vi "PLC_comm.vi"() -> ()   [LabVIEW 2017]
uses:
  <vilib>/addons/database/NI_Database_API.lvlib
  Global/DATA LOG.vi
  Global/Global 1.vi
  <vilib>/DATA AHEAD/SP7/typedefs/PLC Type.ctl
  <vilib>/DATA AHEAD/SP7/SP7.lvlib
  <vilib>/DATA AHEAD/SP7/functions/read/read String.vi
  <vilib>/DATA AHEAD/SP7/functions/write/write Dint array.vi
  <vilib>/DATA AHEAD/SP7/functions/read/read Dint array.vi
  <vilib>/Utility/error.llb/DialogType.ctl
  <vilib>/DATA AHEAD/SP7/functions/read/read real array.vi
  <vilib>/DATA AHEAD/SP7/functions/write/writeString.vi
  <vilib>/addons/database/Connection.llb/DB Tools Open Connec (String).vi
panel:
  out "IP1 7":string
  out "PLC 7":bool
  out "IP1 6":string
  out "PLC 6":bool
  out "IP1 5":string
  out "PLC 5":bool
  out "PLC 4":bool
  out "PLC 3":bool
  out "PLC 2":bool
  out "PLC 1":bool
  out "IP1 4":string
  out "IP1 3":string
  out "IP1 2":string
  out "IP1":string
  in  "stop":bool
  out "error out":errorcluster
  in  "error in (no error)":errorcluster
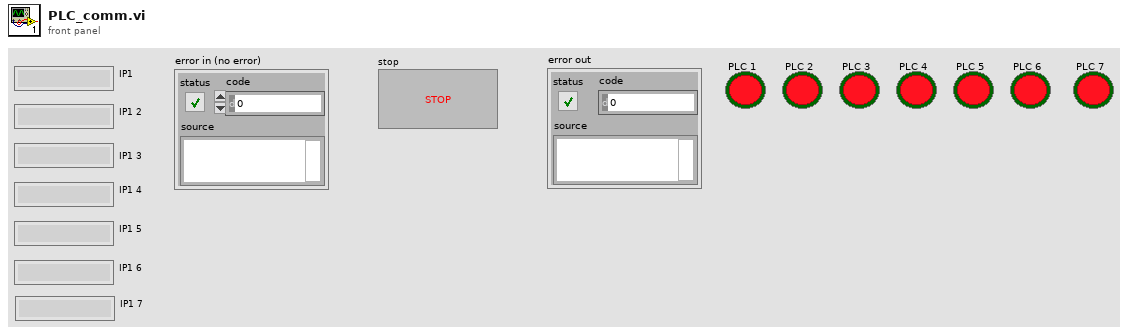
[diagram p1: front panel]
types:
  T1 = typedef "DialogType.ctl" = u16
  T2 = typedef "SP7.lvlib/PLC Type.ctl" = enum16{"S7 200", "S7 300/400", "S7 1200", "S7 1500", "LOGO!8"}
  T3 = typedef "NI_Database_API.lvlib/Conn ObjectReference.ctl" = refnum<k1>
  T4 = typedef "SP7.lvlib/S7 Connection.ctl" = cluster{"TCP Connection Ref":refnum<k5>, "IP address":string, "timeout ms":i32, "Connected?":bool, "PLC Type":T2, "Rack S7 400":u8, "Slot S7 400":u8, "PDU Size":u16, "connection semaphore":T5}
  T5 = typedef "Semaphore RefNum" = refnum<k1>
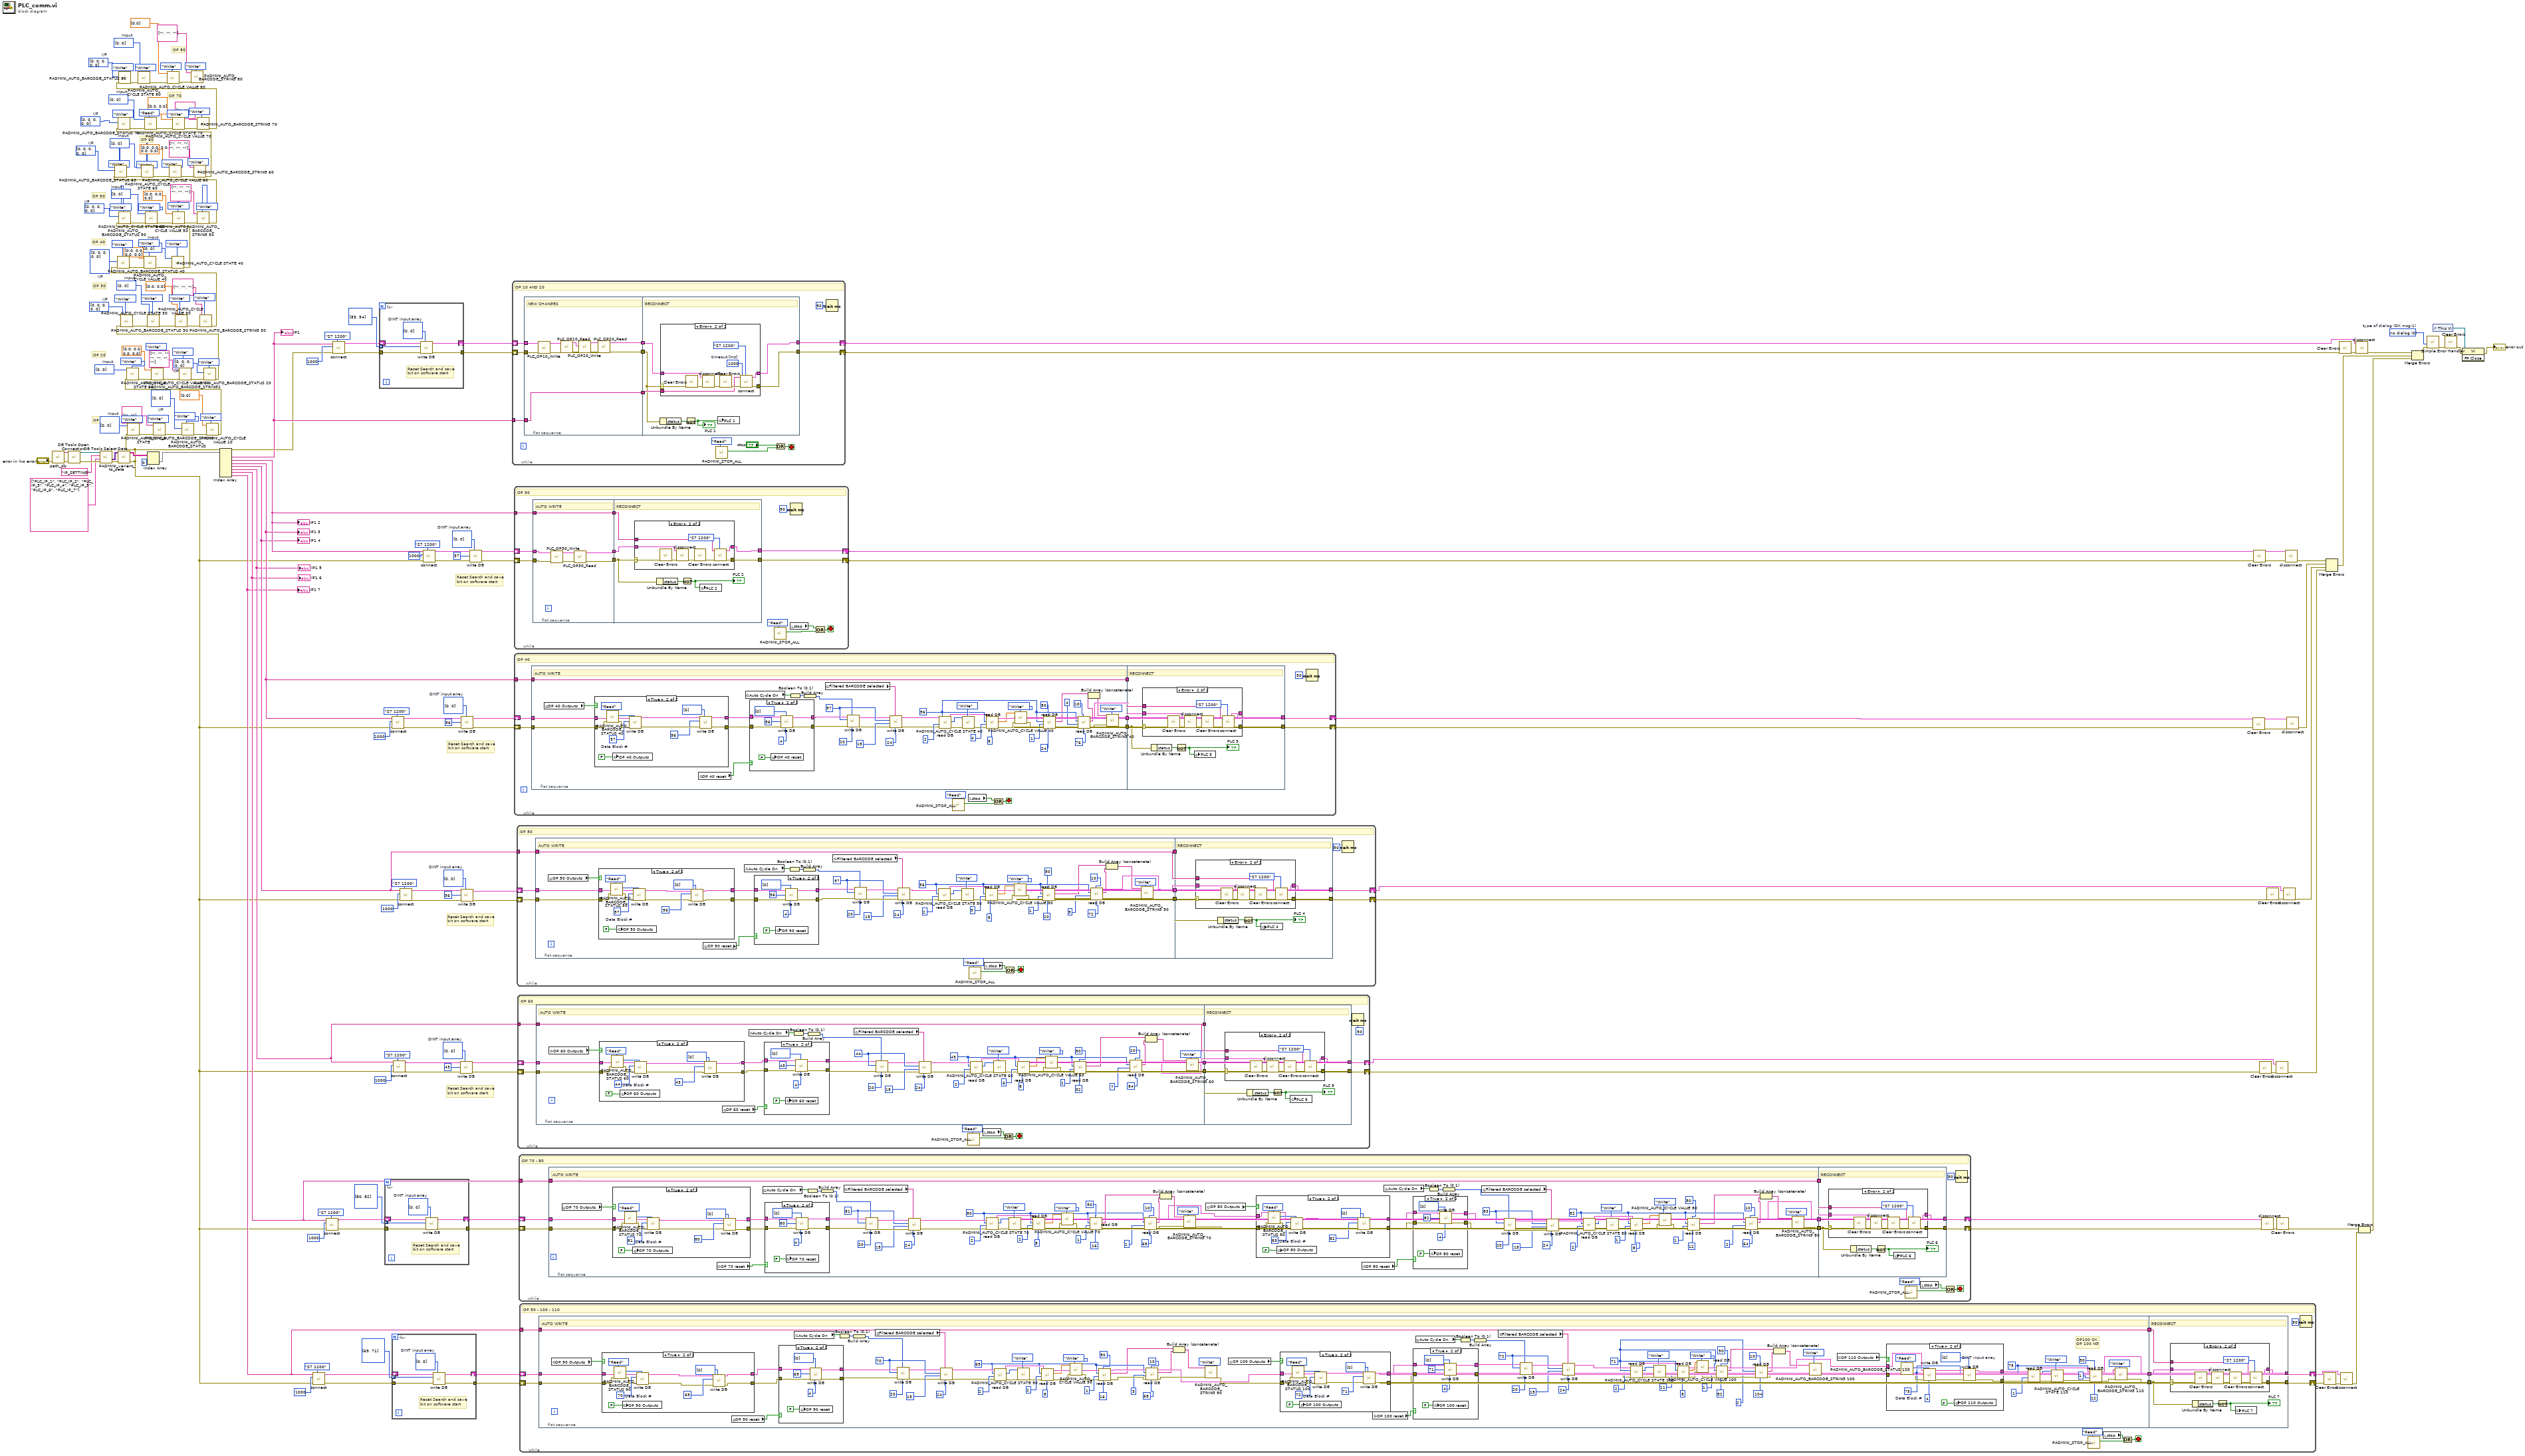
[diagram p0: block diagram]
diagram:
  w15 = i32[] [0, 0]  # DINT input array
  w22 = i32[] [0, 0]  # DINT input array
  w27 = i32[] [0, 0]  # DINT input array
  w39 = i32[] [0, 0]  # DINT input array
  w40 = T1 0 items=["no dialog", "OK message", "continue or stop message", "OK message + warnings", "continue/stop + warnings"]  # type of dialog (OK msg:1)
  w42 = i32[] [0, 0, 0, 0, 0]  # I/P
  w43 = i32[] [0, 0]  # Input
  w45 = i32[] [0, 0]  # Input
  w46 = i32[] [0, 0]  # Input
  w48 = i32[] [0, 0]  # Input
  w44 = i32[] [0, 0, 0, 0, 0]  # I/P
  w47 = i32[] [0, 0, 0, 0, 0]  # I/P
  w49 = i32[] [0, 0, 0, 0, 0]  # I/P
  w50 = i32[] [0, 0, 0, 0, 0]  # I/P
  w51 = i32[] [0, 0]  # Input
  w52 = i32[] [0, 0]  # Input
  w53 = i32[] [0, 0, 0, 0, 0]  # I/P
  w54 = i32[] [0, 0, 0, 0, 0]  # I/P
  w55 = i32[] [0, 0]  # Input
  w56 = i32[] [0, 0]  # I/P
  w57 = i32[] [0, 0]  # Input
  # "Reset Search and save \nbit on software start"
  # "Reset Search and save \nbit on software start"
  # "Reset Search and save \nbit on software start"
  # "Reset Search and save \nbit on software start"
  # "OP 80"
  # "OP 70"
  # "OP 60"
  # "OP 50"
  # "OP 40"
  # "OP 30"
  # "OP 20"
  # "OP 10"
  n1 = call "path_db.vi"("error in"="error in (no error)") -> ("error out"=w196:errorcluster, "resulting string"=w201:string)  [unwired: 9 in]
  n2 = call-poly <vilib>:"DB Tools Open Connection.vi"("error in (no error)"=w196, "connection information"=w201) -> ("error out"=w200:errorcluster, "connection reference"=w199:T3)  [unwired: 6 in]
  n3 = call <vilib>:"DB Tools Select Data.vi"("error in (no error)"=w200, "columns"=string[] ["PLC_IP_1", "PLC_IP_2", "PLC_IP_3", "PLC_IP_4", "PLC_IP_5", "PLC_IP_6", "PLC_IP_7"], "table"="IP_SETTING", "connection reference"=w199) -> ("error out"=w198:errorcluster, "data"=w197:variant[][])  [unwired: 2 in, 1 out]
  n4 = call "PADMINI_varient_to_data.vi"("error in (no error)"=w198, "data"=w197) -> ("error out"=w64:errorcluster, "Array"=w192:string[][])  [unwired: 8 in]
  n5 = call "PADMINI_AUTO_CYCLE STATE.vi"("Enum"=enum16{"Read", "Write"}."Write", "error in (no error)"=w64, "Input"=w57) -> ("error out"=w180:errorcluster)  [unwired: 7 in, 1 out]
  n6 = Index Array(array=w192, index (row)=0) -> (element=w191:string[])  [unwired: 1 in]
  n7 = call "PADMINI_AUTO_BARCODE_STRING.vi"("Enum"=enum16{"Read", "Write"}."Write", "error in (no error)"=w180, "Input"=string[] ["", ""]) -> ("error out"=w177:errorcluster)  [unwired: 7 in, 1 out]
  n8 = call "PADMINI_AUTO_BARCODE_STATUS.vi"("Enum"=enum16{"Read", "Write"}."Write", "error in (no error)"=w177, "I/P"=w56) -> ("error out"=w175:errorcluster)  [unwired: 7 in, 1 out]
  n9 = call "PADMINI_AUTO_CYCLE VALUE 10.vi"("Enum"=enum16{"Read", "Write"}."Write", "error in (no error)"=w175, "Input"=dbl[] [0.0]) -> ("error out"=w169:errorcluster)  [unwired: 7 in, 1 out]
  n10 = call "PADMINI_AUTO_CYCLE STATE 20.vi"("Enum"=enum16{"Read", "Write"}."Write", "error in (no error)"=w169, "Input"=w43) -> ("error out"=w167:errorcluster)  [unwired: 7 in, 1 out]
  n11 = call "PADMINI_AUTO_CYCLE VALUE 20.vi"("Enum"=enum16{"Read", "Write"}."Write", "error in (no error)"=w167, "Input"=dbl[] [0.0, 0.0, 0.0, 0.0]) -> ("error out"=w163:errorcluster)  [unwired: 7 in, 1 out]
  n12 = call "PADMINI_AUTO_BARCODE_STRING2.vi"("Enum"=enum16{"Read", "Write"}."Write", "error in (no error)"=w163, "Input"=string[] ["", "", "", "", "", "", ""]) -> ("error out"=w161:errorcluster)  [unwired: 7 in, 1 out]
  n13 = call "PADMINI_AUTO_BARCODE_STATUS 20.vi"("Enum"=enum16{"Read", "Write"}."Write", "error in (no error)"=w161, "I/P"=w42) -> ("error out"=w157:errorcluster)  [unwired: 7 in, 1 out]
  n14 = call "PADMINI_AUTO_BARCODE_STATUS 30.vi"("Enum"=enum16{"Read", "Write"}."Write", "error in (no error)"=w157, "I/P"=w44) -> ("error out"=w154:errorcluster)  [unwired: 7 in, 1 out]
  n15 = call "PADMINI_AUTO_CYCLE STATE 30.vi"("Enum"=enum16{"Read", "Write"}."Write", "error in (no error)"=w154, "Input"=w45) -> ("error out"=w153:errorcluster)  [unwired: 7 in, 1 out]
  n16 = call "PADMINI_AUTO_CYCLE VALUE 30.vi"("Enum"=enum16{"Read", "Write"}."Write", "error in (no error)"=w153, "Input"=dbl[] [0.0, 0.0]) -> ("error out"=w150:errorcluster)  [unwired: 7 in, 1 out]
  n17 = call "PADMINI_AUTO_BARCODE_STRING 30.vi"("Enum"=enum16{"Read", "Write"}."Write", "error in (no error)"=w150, "Input"=string[] ["", "", ""]) -> ("error out"=w131:errorcluster)  [unwired: 7 in, 1 out]
  n18 = call "PADMINI_AUTO_BARCODE_STATUS 40.vi"("Enum"=enum16{"Read", "Write"}."Write", "error in (no error)"=w131, "I/P"=w47) -> ("error out"=w130:errorcluster)  [unwired: 7 in, 1 out]
  n19 = call "PADMINI_AUTO_CYCLE VALUE 40.vi"("Enum"=enum16{"Read", "Write"}."Write", "error in (no error)"=w130, "Input"=dbl[] [0.0, 0.0, 0.0, 0.0]) -> ("error out"=w129:errorcluster)  [unwired: 7 in, 1 out]
  n20 = call "PADMINI_AUTO_CYCLE STATE 40.vi"("Enum"=enum16{"Read", "Write"}."Write", "error in (no error)"=w129, "Input"=w46) -> ("error out"=w128:errorcluster)  [unwired: 7 in, 1 out]
  n21 = call "PADMINI_AUTO_BARCODE_STATUS 50.vi"("Enum"=enum16{"Read", "Write"}."Write", "error in (no error)"=w128, "I/P"=w49) -> ("error out"=w115:errorcluster)  [unwired: 7 in, 1 out]
  n22 = call "PADMINI_AUTO_CYCLE STATE 50.vi"("Enum"=enum16{"Read", "Write"}."Write", "error in (no error)"=w115, "Input"=w48) -> ("error out"=w119:errorcluster)  [unwired: 7 in, 1 out]
  n23 = call "PADMINI_AUTO_CYCLE VALUE 50.vi"("Enum"=enum16{"Read", "Write"}."Write", "error in (no error)"=w119, "Input"=dbl[] [0.0, 0.0, 0.0]) -> ("error out"=w116:errorcluster)  [unwired: 7 in, 1 out]
  n24 = call "PADMINI_AUTO_BARCODE_STRING 50.vi"("Enum"=enum16{"Read", "Write"}."Write", "error in (no error)"=w116, "Input"=string[] ["", "", "", "", "", ""]) -> ("error out"=w94:errorcluster)  [unwired: 7 in, 1 out]
  n25 = call "PADMINI_AUTO_BARCODE_STATUS 60.vi"("Enum"=enum16{"Read", "Write"}."Write", "error in (no error)"=w94, "I/P"=w50) -> ("error out"=w98:errorcluster)  [unwired: 7 in, 1 out]
  n26 = call "PADMINI_AUTO_CYCLE STATE 60.vi"("Enum"=enum16{"Read", "Write"}."Write", "error in (no error)"=w98, "Input"=w51) -> ("error out"=w100:errorcluster)  [unwired: 7 in, 1 out]
  n27 = call "PADMINI_AUTO_CYCLE VALUE 60.vi"("Enum"=enum16{"Read", "Write"}."Write", "error in (no error)"=w100, "Input"=dbl[] [0.0, 0.0, 0.0, 0.0, 0.0]) -> ("error out"=w103:errorcluster)  [unwired: 7 in, 1 out]
  n28 = call "PADMINI_AUTO_BARCODE_STRING 60.vi"("Enum"=enum16{"Read", "Write"}."Write", "error in (no error)"=w103, "Input"=string[] ["", "", "", "", "", ""]) -> ("error out"=w72:errorcluster)  [unwired: 7 in, 1 out]
  n29 = call "PADMINI_AUTO_BARCODE_STATUS 70.vi"("Enum"=enum16{"Read", "Write"}."Write", "error in (no error)"=w72, "I/P"=w53) -> ("error out"=w75:errorcluster)  [unwired: 7 in, 1 out]
  n30 = call "PADMINI_AUTO_CYCLE STATE 70.vi"("Enum"=enum16{"Read", "Write"}."Read", "error in (no error)"=w75, "Input"=w52) -> ("error out"=w87:errorcluster)  [unwired: 7 in, 1 out]
  n31 = call "PADMINI_AUTO_CYCLE VALUE 70.vi"("Enum"=enum16{"Read", "Write"}."Write", "error in (no error)"=w87, "Input"=dbl[] [0.0, 0.0]) -> ("error out"=w84:errorcluster)  [unwired: 7 in, 1 out]
  n32 = call "PADMINI_AUTO_BARCODE_STRING 70.vi"("Enum"=enum16{"Read", "Write"}."Write", "error in (no error)"=w84, "Input"=string[] ["", ""]) -> ("error out"=w69:errorcluster)  [unwired: 7 in, 1 out]
  n33 = call "PADMINI_AUTO_BARCODE_STATUS 80.vi"("Enum"=enum16{"Read", "Write"}."Write", "error in (no error)"=w69, "I/P"=w54) -> ("error out"=w76:errorcluster)  [unwired: 7 in, 1 out]
  n34 = call "PADMINI_AUTO_CYCLE STATE 80.vi"("Enum"=enum16{"Read", "Write"}."Write", "error in (no error)"=w76, "Input"=w55) -> ("error out"=w80:errorcluster)  [unwired: 7 in, 1 out]
  n35 = call "PADMINI_AUTO_CYCLE VALUE 80.vi"("Enum"=enum16{"Read", "Write"}."Write", "error in (no error)"=w80, "Input"=sgl[] [0.0]) -> ("error out"=w83:errorcluster)  [unwired: 7 in, 1 out]
  n36 = call "PADMINI_AUTO_BARCODE_STRING 80.vi"("Enum"=enum16{"Read", "Write"}."Write", "error in (no error)"=w83, "Input"=string[] ["", "", ""]) -> ()  [unwired: 7 in, 2 out]
  n37 = Index Array(array=w191) -> (element #1=w144:string, element #2=w145:string, element #3=w141:string, element #4=w121:string, element #5=w106:string, element #6=w66:string, element #7=w65:string)  [unwired: 7 in]
  "IP1" <- w144
  "IP1 2" <- w145
  "IP1 3" <- w141
  "IP1 4" <- w121
  "IP1 5" <- w106
  "IP1 6" <- w66
  "IP1 7" <- w65
  n38 = call <vilib>:"connect.vi"("PLC Type"=PLC_Type."S7 1200" ("PLC Type 2"), "error in (no error)"=w64, "timeout [ms]"=1000 ("timeout [ms] 2"), "IP address"=w65) -> ("error out"=w2:errorcluster, "S7 Connection out"=w1:T4)  [unwired: 6 in]
  n39 = call <vilib>:"connect.vi"("PLC Type"=PLC_Type."S7 1200" ("PLC Type 2"), "error in (no error)"=w64, "timeout [ms]"=1000 ("timeout [ms] 2"), "IP address"=w66) -> ("error out"=w6:errorcluster, "S7 Connection out"=w7:T4)  [unwired: 6 in]
  n40 = call <vilib>:"connect.vi"("PLC Type"=PLC_Type."S7 1200" ("PLC Type 2"), "error in (no error)"=w64, "timeout [ms]"=1000, "IP address"=w144) -> ("error out"=w30:errorcluster, "S7 Connection out"=w29:T4)  [unwired: 6 in]
  n41 = for {
    tunnel: u16[] [83, 94] ("Data Block #") -> [w207] mode=indexing
    shift-right: [w205] -> w32
    shift-left: w29 -> [w202]
    tunnel: w30 -> [w203]
    tunnel: [w204] -> w31
    w206 = i32[] [0, 0]  # DINT input array
    # "Reset Search and save \nbit on software start"
    n42 = call-poly <vilib>:"write DB.vi"("DINT input array"=w206, "error in (no error)"=w203, "Data Block #"=w207, "S7 Connection in"=w202) -> ("error out"=w204:errorcluster, "S7 Connection out"=w205:T4)  [unwired: 4 in, 2 out]
  }
  n43 = for {
    tunnel: u16[] [80, 82] ("Data Block #") -> [w213] mode=indexing
    shift-right: [w211] -> w8
    shift-left: w7 -> [w208]
    tunnel: w6 -> [w209]
    tunnel: [w210] -> w9
    w212 = i32[] [0, 0]  # DINT input array
    # "Reset Search and save \nbit on software start"
    n44 = call-poly <vilib>:"write DB.vi"("DINT input array"=w212, "error in (no error)"=w209, "Data Block #"=w213, "S7 Connection in"=w208) -> ("error out"=w210:errorcluster, "S7 Connection out"=w211:T4)  [unwired: 4 in, 2 out]
  }
  n45 = call <vilib>:"connect.vi"("PLC Type"=PLC_Type."S7 1200" ("PLC Type 2"), "error in (no error)"=w64, "timeout [ms]"=1000 ("timeout [ms] 2"), "IP address"=w141) -> ("error out"=w24:errorcluster, "S7 Connection out"=w23:T4)  [unwired: 6 in]
  n46 = for {
    tunnel: u16[] [69, 71] ("Data Block #") -> [w219] mode=indexing
    shift-right: [w217] -> w4
    shift-left: w1 -> [w214]
    tunnel: w2 -> [w215]
    tunnel: [w216] -> w3
    w218 = i32[] [0, 0]  # DINT input array
    # "Reset Search and save \nbit on software start"
    n47 = call-poly <vilib>:"write DB.vi"("DINT input array"=w218, "error in (no error)"=w215, "Data Block #"=w219, "S7 Connection in"=w214) -> ("error out"=w216:errorcluster, "S7 Connection out"=w217:T4)  [unwired: 4 in, 2 out]
  }
  n48 = call <vilib>:"connect.vi"("PLC Type"=PLC_Type."S7 1200" ("PLC Type 2"), "error in (no error)"=w64, "timeout [ms]"=1000 ("timeout [ms] 2"), "IP address"=w106) -> ("error out"=w11:errorcluster, "S7 Connection out"=w12:T4)  [unwired: 6 in]
  n49 = call <vilib>:"connect.vi"("PLC Type"=PLC_Type."S7 1200" ("PLC Type 2"), "error in (no error)"=w64, "timeout [ms]"=1000 ("timeout [ms] 2"), "IP address"=w121) -> ("error out"=w18:errorcluster, "S7 Connection out"=w17:T4)  [unwired: 6 in]
  n50 = call <vilib>:"connect.vi"("PLC Type"=PLC_Type."S7 1200" ("PLC Type 2"), "error in (no error)"=w64, "timeout [ms]"=1000 ("timeout [ms] 2"), "IP address"=w145) -> ("error out"=w36:errorcluster, "S7 Connection out"=w37:T4)  [unwired: 6 in]
  n51 = call-poly <vilib>:"write DB.vi"("DINT input array"=w15, "error in (no error)"=w11, "Data Block #"=u16 43, "S7 Connection in"=w12) -> ("error out"=w14:errorcluster, "S7 Connection out"=w13:T4)  [unwired: 4 in, 2 out]
  n52 = call-poly <vilib>:"write DB.vi"("DINT input array"=w22, "error in (no error)"=w18, "Data Block #"=u16 56, "S7 Connection in"=w17) -> ("error out"=w19:errorcluster, "S7 Connection out"=w20:T4)  [unwired: 4 in, 2 out]
  n53 = call-poly <vilib>:"write DB.vi"("DINT input array"=w27, "error in (no error)"=w24, "Data Block #"=u16 56, "S7 Connection in"=w23) -> ("error out"=w26:errorcluster, "S7 Connection out"=w25:T4)  [unwired: 4 in, 2 out]
  n54 = call-poly <vilib>:"write DB.vi"("DINT input array"=w39, "error in (no error)"=w36, "Data Block #"=u16 37, "S7 Connection in"=w37) -> ("error out"=w35:errorcluster, "S7 Connection out"=w34:T4)  [unwired: 4 in, 2 out]
  n55 = while {
    shift-right: [w222] -> w172
    shift-left: w32 -> [w232]
    shift-right: [w230] -> w185
    shift-left: w31 -> [w231]
    tunnel: w144 -> [w220]
    stop <- w225 stop-if-true
    # "OP 10 AND 20"
    n56 = flat-sequence {
      tunnel: [w235] -> w224
      tunnel: [w241] -> w223
      tunnel: w231 -> [w242]
      tunnel: w232 -> [w243]
      tunnel: [w240] -> w221
      tunnel: w220 -> [w240]
      tunnel: [w247] -> w230
      tunnel: [w246] -> w222
      tunnel: w224 -> [w248]
      tunnel: w223 -> [w244]
      tunnel: w221 -> [w245]
      frame #0 {
        # "NEW CHANGES"
        n57 = call "PLC_OP10_Write.vi"("error in (no error)"=w242, "S7 Connection in"=w243) -> ("error out"=w238:errorcluster, "S7 Connection out"=w239:T4)  [unwired: 8 in]
        n58 = call "PLC_OP10_Read.vi"("error in (no error)"=w238, "S7 Connection in"=w239) -> ("error out"=w237:errorcluster, "S7 Connection out"=w236:T4)  [unwired: 8 in]
        n59 = call "PLC_OP20_Write.vi"("error in (no error)"=w237, "S7 Connection in"=w236) -> ("error out"=w233:errorcluster, "S7 Connection out"=w234:T4)  [unwired: 8 in]
        n60 = call "PLC_OP20_Read.vi"("error in (no error)"=w233, "S7 Connection in"=w234) -> ("error out"=w241:errorcluster, "S7 Connection out 2"=w235:T4)  [unwired: 8 in]
      }
      frame #1 {
        # "RECONNECT"
        n61 = Unbundle By Name(w244) -> ("status"=w250:bool)
        n62 = case shown="Error" w244 {
          selector: w244 -> [w252 w261]
          tunnel: [w251 w258] -> w246
          tunnel: [w252 w259] -> w247
          tunnel: w248 -> [w251 w255]
          tunnel: w245 -> [_ w254]
          frame No Error {
          }
          frame Error {
            w253 = 1000  # timeout [ms]
            n63 = call <vilib>:"Clear Errors.vi"("error in (no error)"=w261) -> ("error out"=w262:errorcluster)  [unwired: 5 in, 1 out]
            n64 = call <vilib>:"disconnect.vi"("error in (no error)"=w262, "S7 Connection in"=w255) -> ("error out"=w260:errorcluster)  [unwired: 8 in, 1 out]
            n65 = call <vilib>:"Clear Errors.vi"("error in (no error)"=w260) -> ("error out"=w257:errorcluster)  [unwired: 5 in, 1 out]
            n66 = call <vilib>:"connect.vi"("PLC Type"=PLC_Type."S7 1200" ("PLC Type 2"), "error in (no error)"=w257, "timeout [ms]"=w253, "IP address"=w254) -> ("error out"=w259:errorcluster, "S7 Connection out"=w258:T4)  [unwired: 6 in]
          }
        }
        n67 = Not(x=w250) -> (.not. x?=w249:bool)
        "PLC 1" <- w249
        n68 = global write "Global 1.vi" "PLC 1"(w249) -> ()
      }
    }
    n69 = call "PADMINI_STOP_ALL.vi"("Enum"=enum16{"Read", "Write"}."Read") -> ("Boolean 2"=w227:bool)  [unwired: 9 in, 1 out]
    n70 = Or(x="stop", y=w227) -> (x .or. y?=w225:bool)
    n71 = Wait (ms)(milliseconds to wait=u32 50) -> ()  [unwired: 1 out]
  }
  n72 = while {
    shift-right: [w265] -> w147
    shift-left: w34 -> [w275]
    shift-right: [w273] -> w146
    shift-left: w35 -> [w274]
    tunnel: w145 -> [w264]
    stop <- w267 stop-if-true
    # "OP 30"
    n73 = flat-sequence {
      tunnel: [w278] -> w271
      tunnel: [w280] -> w266
      tunnel: w274 -> [w282]
      tunnel: w275 -> [w281]
      tunnel: w264 -> [w279]
      tunnel: [w279] -> w263
      tunnel: [w285] -> w273
      tunnel: [w284] -> w265
      tunnel: w271 -> [w287]
      tunnel: w266 -> [w286]
      tunnel: w263 -> [w283]
      frame #0 {
        # "AUTO WRITE"
        n74 = call "PLC_OP30_Write.vi"("error in (no error)"=w282, "S7 Connection in"=w281) -> ("error out"=w276:errorcluster, "S7 Connection out"=w277:T4)  [unwired: 8 in]
        n75 = call "PLC_OP30_Read.vi"("error in (no error)"=w276, "S7 Connection in"=w277) -> ("error out"=w280:errorcluster, "S7 Connection out 2"=w278:T4)  [unwired: 8 in]
      }
      frame #1 {
        # "RECONNECT"
        n76 = case shown="Error" w286 {
          selector: w286 -> [w291 w299]
          tunnel: [w290 w296] -> w284
          tunnel: [w291 w297] -> w285
          tunnel: w287 -> [w290 w293]
          tunnel: w283 -> [_ w292]
          frame No Error {
          }
          frame Error {
            n77 = call <vilib>:"Clear Errors.vi"("error in (no error)"=w299) -> ("error out"=w300:errorcluster)  [unwired: 5 in, 1 out]
            n78 = call <vilib>:"disconnect.vi"("error in (no error)"=w300, "S7 Connection in"=w293) -> ("error out"=w298:errorcluster)  [unwired: 8 in, 1 out]
            n79 = call <vilib>:"Clear Errors.vi"("error in (no error)"=w298) -> ("error out"=w295:errorcluster)  [unwired: 5 in, 1 out]
            n80 = call <vilib>:"connect.vi"("PLC Type"=PLC_Type."S7 1200" ("PLC Type 2"), "error in (no error)"=w295, "IP address"=w292) -> ("error out"=w297:errorcluster, "S7 Connection out"=w296:T4)  [unwired: 7 in]
          }
        }
        n81 = Unbundle By Name(w286) -> ("status"=w289:bool)
        n82 = Not(x=w289) -> (.not. x?=w288:bool)
        "PLC 2" <- w288
        n83 = global write "Global 1.vi" "PLC 2"(w288) -> ()
      }
    }
    n84 = call "PADMINI_STOP_ALL.vi"("Enum"=enum16{"Read", "Write"}."Read") -> ("Boolean 2"=w269:bool)  [unwired: 9 in, 1 out]
    n85 = Wait (ms)(milliseconds to wait=u32 50) -> ()  [unwired: 1 out]
    n86 = local read "stop"() -> (w268:bool)
    n87 = Or(x=w268, y=w269) -> (x .or. y?=w267:bool)
  }
  n88 = while {
    shift-right: [w303] -> w138
    shift-left: w25 -> [w313]
    shift-right: [w311] -> w139
    shift-left: w26 -> [w312]
    tunnel: w141 -> [w302]
    stop <- w305 stop-if-true
    # "OP 40"
    n89 = flat-sequence {
      tunnel: [w325] -> w309
      tunnel: [w344] -> w304
      tunnel: w312 -> [w363]
      tunnel: w313 -> [w362]
      tunnel: w302 -> [w343]
      tunnel: [w343] -> w301
      tunnel: [w391] -> w311
      tunnel: [w390] -> w303
      tunnel: w309 -> [w393]
      tunnel: w304 -> [w392]
      tunnel: w301 -> [w389]
      frame #0 {
        w336 = u16 57 ("Data Block #")
        w324 = u16 56 ("Data Block #")
        # "AUTO WRITE"
        n90 = global read "DATA LOG.vi" "OP 40 Outputs"() -> (w361:bool)
        n91 = case shown="True" w361 {
          tunnel: w362 -> [w374 w387]
          tunnel: [w375 w379] -> w341
          tunnel: [w374 w381] -> w342
          tunnel: w363 -> [w375 w384]
          frame False {
          }
          frame True {
            w388 = u16 57  # Data Block #
            n92 = call "PADMINI_AUTO_BARCODE_STATUS 40.vi"("Enum"=enum16{"Read", "Write"}."Read", "error in (no error)"=w384) -> ("error out"=w383:errorcluster, "O/P"=w385:i32[])  [unwired: 8 in]
            n93 = global write "DATA LOG.vi" "OP 40 Outputs"(FALSE) -> ()
            n94 = call-poly <vilib>:"write DB.vi"("DINT input array"=w385, "error in (no error)"=w383, "Data Block #"=w388, "S7 Connection in"=w387) -> ("error out"=w378:errorcluster, "S7 Connection out"=w380:T4)  [unwired: 4 in, 2 out]
            n95 = call-poly <vilib>:"write DB.vi"("DINT input array"=i32[] [0], "error in (no error)"=w378, "Data Block #"=u16 56, "S7 Connection in"=w380) -> ("error out"=w379:errorcluster, "S7 Connection out"=w381:T4)  [unwired: 4 in, 2 out]
          }
        }
        n96 = global read "DATA LOG.vi" "OP 40 reset"() -> (w340:bool)
        n97 = global read "DATA LOG.vi" "Auto Cycle On"() -> (w316:bool)
        n98 = case shown="True" w340 {
          tunnel: w341 -> [w364 w373]
          tunnel: [w364 w372] -> w329
          tunnel: w342 -> [w365 w371]
          tunnel: [w365 w370] -> w330
          frame False {
          }
          frame True {
            n99 = global write "DATA LOG.vi" "OP 40 reset"(FALSE) -> ()
            n100 = call-poly <vilib>:"write DB.vi"("Item offset [byte]"=u16 4 ("Data Block #"), "DINT input array"=i32[] [0], "error in (no error)"=w373, "Data Block #"=u16 56, "S7 Connection in"=w371) -> ("error out"=w372:errorcluster, "S7 Connection out"=w370:T4)  [unwired: 3 in, 2 out]
          }
        }
        n101 = Boolean To (0,1)(Boolean=w316) -> (0, 1=w315:i16)
        n102 = Build Array(w315) -> (w314:i16[])
        n103 = global read "Global 1.vi" "Filtered BARCODE selected"() -> (w339:string[])
        n104 = call-poly <vilib>:"write DB.vi"("Item offset [byte]"=u32 20, "DINT input array"=w314, "error in (no error)"=w329, "Data Block #"=w336, "S7 Connection in"=w330) -> ("error out"=w334:errorcluster, "S7 Connection out"=w333:T4)  [unwired: 3 in, 2 out]
        n105 = call-poly <vilib>:"write DB.vi"("Item offset [byte]"=u32 24, "Input STRINGS"=w339, "error in (no error)"=w334, "String length reserved in DB (default=254)"=u16 15, "Data Block #"=w336, "S7 Connection in"=w333) -> ("error out"=w331:errorcluster, "S7 Connection out"=w332:T4)  [unwired: 2 in, 2 out]
        n106 = call-poly <vilib>:"read DB.vi"("error in (no error)"=w331, "items #"=u16 2 ("Items # [byte]"), "Data Block #"=w324, "S7 Connection in"=w332) -> ("error out"=w359:errorcluster, "DINT result array"=w357:i32[], "S7 Connection out"=w354:T4)  [unwired: 5 in]
        n107 = call "PADMINI_AUTO_CYCLE STATE 40.vi"("Enum"=enum16{"Read", "Write"}."Write", "error in (no error)"=w359, "Input"=w357) -> ("error out"=w355:errorcluster)  [unwired: 7 in, 1 out]
        n108 = call-poly <vilib>:"read DB.vi"("Item offset [byte]"=u32 8, "error in (no error)"=w355, "items #"=u16 4 ("Items # [byte]"), "Data Block #"=w324, "S7 Connection in"=w354) -> ("error out"=w347:errorcluster, "REAL result array"=w345:sgl[], "S7 Connection out"=w353:T4)  [unwired: 4 in]
        n109 = call "PADMINI_AUTO_CYCLE VALUE 40.vi"("Enum"=enum16{"Read", "Write"}."Write", "error in (no error)"=w347, "Input"=w345) -> ("error out"=w346:errorcluster)  [unwired: 7 in, 1 out]
        n110 = call-poly <vilib>:"read DB.vi"("Item offset [byte]"=u32 24, "String length reserved in DB (default=254)"=u16 50, "error in (no error)"=w346, "items #"=u16 1 ("Items # [byte]"), "Data Block #"=w324, "S7 Connection in"=w353) -> ("error out"=w328:errorcluster, "STRING result Array"=w319:string[], "S7 Connection out"=w326:T4)  [unwired: 2 in, 1 out]
        n111 = call-poly <vilib>:"read DB.vi"("Item offset [byte]"=u32 76, "String length reserved in DB (default=254)"=u16 10, "error in (no error)"=w328, "items #"=u16 4 ("Items # [byte]"), "Data Block #"=w324, "S7 Connection in"=w326) -> ("error out"=w327:errorcluster, "STRING result Array"=w318:string[], "S7 Connection out"=w325:T4)  [unwired: 2 in, 1 out]
        n112 = Build Array (concatenate)(w319, w318) -> (w317:string[])
        n113 = call "PADMINI_AUTO_BARCODE_STRING 40.vi"("Enum"=enum16{"Read", "Write"}."Write", "error in (no error)"=w327, "Input"=w317) -> ("error out"=w344:errorcluster)  [unwired: 7 in, 1 out]
      }
      frame #1 {
        # "RECONNECT"
        n114 = case shown="Error" w392 {
          selector: w392 -> [w397 w405]
          tunnel: [w396 w402] -> w390
          tunnel: [w397 w403] -> w391
          tunnel: w393 -> [w396 w399]
          tunnel: w389 -> [_ w398]
          frame No Error {
          }
          frame Error {
            n115 = call <vilib>:"Clear Errors.vi"("error in (no error)"=w405) -> ("error out"=w406:errorcluster)  [unwired: 5 in, 1 out]
            n116 = call <vilib>:"disconnect.vi"("error in (no error)"=w406, "S7 Connection in"=w399) -> ("error out"=w404:errorcluster)  [unwired: 8 in, 1 out]
            n117 = call <vilib>:"Clear Errors.vi"("error in (no error)"=w404) -> ("error out"=w401:errorcluster)  [unwired: 5 in, 1 out]
            n118 = call <vilib>:"connect.vi"("PLC Type"=PLC_Type."S7 1200" ("PLC Type 2"), "error in (no error)"=w401, "IP address"=w398) -> ("error out"=w403:errorcluster, "S7 Connection out"=w402:T4)  [unwired: 7 in]
          }
        }
        n119 = Unbundle By Name(w392) -> ("status"=w395:bool)
        n120 = Not(x=w395) -> (.not. x?=w394:bool)
        "PLC 3" <- w394
        n121 = global write "Global 1.vi" "PLC 3"(w394) -> ()
      }
    }
    n122 = call "PADMINI_STOP_ALL.vi"("Enum"=enum16{"Read", "Write"}."Read") -> ("Boolean 2"=w307:bool)  [unwired: 9 in, 1 out]
    n123 = local read "stop"() -> (w306:bool)
    n124 = Or(x=w306, y=w307) -> (x .or. y?=w305:bool)
    n125 = Wait (ms)(milliseconds to wait=u32 50) -> ()  [unwired: 1 out]
  }
  n126 = while {
    shift-right: [w409] -> w126
    shift-left: w20 -> [w419]
    shift-right: [w417] -> w125
    shift-left: w19 -> [w418]
    tunnel: w121 -> [w408]
    stop <- w411 stop-if-true
    # "OP 50"
    n127 = flat-sequence {
      tunnel: [w440] -> w415
      tunnel: [w450] -> w410
      tunnel: w418 -> [w469]
      tunnel: w419 -> [w468]
      tunnel: w408 -> [w449]
      tunnel: [w449] -> w407
      tunnel: [w497] -> w417
      tunnel: [w496] -> w409
      tunnel: w415 -> [w499]
      tunnel: w410 -> [w498]
      tunnel: w407 -> [w495]
      frame #0 {
        w431 = u16 57 ("Data Block #")
        w439 = u16 56 ("Data Block #")
        # "AUTO WRITE"
        n128 = global read "DATA LOG.vi" "OP 50 Outputs"() -> (w467:bool)
        n129 = case shown="True" w467 {
          tunnel: w468 -> [w480 w493]
          tunnel: [w481 w482] -> w448
          tunnel: [w480 w485] -> w447
          tunnel: w469 -> [w481 w490]
          frame False {
          }
          frame True {
            w494 = u16 57  # Data Block #
            n130 = call "PADMINI_AUTO_BARCODE_STATUS 50.vi"("Enum"=enum16{"Read", "Write"}."Read", "error in (no error)"=w490) -> ("error out"=w489:errorcluster, "O/P"=w491:i32[])  [unwired: 8 in]
            n131 = global write "DATA LOG.vi" "OP 50 Outputs"(FALSE) -> ()
            n132 = call-poly <vilib>:"write DB.vi"("DINT input array"=w491, "error in (no error)"=w489, "Data Block #"=w494, "S7 Connection in"=w493) -> ("error out"=w483:errorcluster, "S7 Connection out"=w484:T4)  [unwired: 4 in, 2 out]
            n133 = call-poly <vilib>:"write DB.vi"("DINT input array"=i32[] [0] ("Data Byte"), "error in (no error)"=w483, "Data Block #"=u16 56, "S7 Connection in"=w484) -> ("error out"=w482:errorcluster, "S7 Connection out"=w485:T4)  [unwired: 4 in, 2 out]
          }
        }
        n134 = global read "DATA LOG.vi" "OP 50 reset"() -> (w446:bool)
        n135 = global read "DATA LOG.vi" "Auto Cycle On"() -> (w422:bool)
        n136 = case shown="True" w446 {
          tunnel: w448 -> [w470 w479]
          tunnel: [w470 w478] -> w424
          tunnel: w447 -> [w471 w477]
          tunnel: [w471 w476] -> w427
          frame False {
          }
          frame True {
            n137 = global write "DATA LOG.vi" "OP 50 reset"(FALSE) -> ()
            n138 = call-poly <vilib>:"write DB.vi"("Item offset [byte]"=u16 4 ("Data Block #"), "DINT input array"=i32[] [0], "error in (no error)"=w479, "Data Block #"=u16 56, "S7 Connection in"=w477) -> ("error out"=w478:errorcluster, "S7 Connection out"=w476:T4)  [unwired: 3 in, 2 out]
          }
        }
        n139 = Boolean To (0,1)(Boolean=w422) -> (0, 1=w421:i16)
        n140 = Build Array(w421) -> (w420:i16[])
        n141 = global read "Global 1.vi" "Filtered BARCODE selected"() -> (w428:string[])
        n142 = call-poly <vilib>:"write DB.vi"("Item offset [byte]"=u32 20, "DINT input array"=w420, "error in (no error)"=w424, "Data Block #"=w431, "S7 Connection in"=w427) -> ("error out"=w433:errorcluster, "S7 Connection out"=w434:T4)  [unwired: 3 in, 2 out]
        n143 = call-poly <vilib>:"write DB.vi"("Item offset [byte]"=u32 24, "Input STRINGS"=w428, "error in (no error)"=w433, "String length reserved in DB (default=254)"=u16 15, "Data Block #"=w431, "S7 Connection in"=w434) -> ("error out"=w425:errorcluster, "S7 Connection out"=w426:T4)  [unwired: 2 in, 2 out]
        n144 = call-poly <vilib>:"read DB.vi"("error in (no error)"=w425, "items #"=u16 2 ("Items # [byte]"), "Data Block #"=w439, "S7 Connection in"=w426) -> ("error out"=w465:errorcluster, "DINT result array"=w463:i32[], "S7 Connection out"=w460:T4)  [unwired: 5 in]
        n145 = call "PADMINI_AUTO_CYCLE STATE 50.vi"("Enum"=enum16{"Read", "Write"}."Write", "error in (no error)"=w465, "Input"=w463) -> ("error out"=w461:errorcluster)  [unwired: 7 in, 1 out]
        n146 = call-poly <vilib>:"read DB.vi"("Item offset [byte]"=u32 8, "error in (no error)"=w461, "items #"=u16 3 ("Items # [byte]"), "Data Block #"=w439, "S7 Connection in"=w460) -> ("error out"=w453:errorcluster, "REAL result array"=w451:sgl[], "S7 Connection out"=w459:T4)  [unwired: 4 in]
        n147 = call "PADMINI_AUTO_CYCLE VALUE 50.vi"("Enum"=enum16{"Read", "Write"}."Write", "error in (no error)"=w453, "Input"=w451) -> ("error out"=w452:errorcluster)  [unwired: 7 in, 1 out]
        n148 = call-poly <vilib>:"read DB.vi"("Item offset [byte]"=u32 20, "String length reserved in DB (default=254)"=u16 50, "error in (no error)"=w452, "items #"=u16 1 ("Items # [byte]"), "Data Block #"=w439, "S7 Connection in"=w459) -> ("error out"=w442:errorcluster, "STRING result Array"=w438:string[], "S7 Connection out"=w441:T4)  [unwired: 2 in, 1 out]
        n149 = call-poly <vilib>:"read DB.vi"("Item offset [byte]"=u32 72, "String length reserved in DB (default=254)"=u16 10, "error in (no error)"=w442, "items #"=u16 5 ("Items # [byte]"), "Data Block #"=w439, "S7 Connection in"=w441) -> ("error out"=w443:errorcluster, "STRING result Array"=w437:string[], "S7 Connection out"=w440:T4)  [unwired: 2 in, 1 out]
        n150 = Build Array (concatenate)(w438, w437) -> (w436:string[])
        n151 = call "PADMINI_AUTO_BARCODE_STRING 50.vi"("Enum"=enum16{"Read", "Write"}."Write", "error in (no error)"=w443, "Input"=w436) -> ("error out"=w450:errorcluster)  [unwired: 7 in, 1 out]
      }
      frame #1 {
        # "RECONNECT"
        n152 = case shown="Error" w498 {
          selector: w498 -> [w503 w511]
          tunnel: [w502 w508] -> w496
          tunnel: [w503 w509] -> w497
          tunnel: w499 -> [w502 w505]
          tunnel: w495 -> [_ w504]
          frame No Error {
          }
          frame Error {
            n153 = call <vilib>:"Clear Errors.vi"("error in (no error)"=w511) -> ("error out"=w512:errorcluster)  [unwired: 5 in, 1 out]
            n154 = call <vilib>:"disconnect.vi"("error in (no error)"=w512, "S7 Connection in"=w505) -> ("error out"=w510:errorcluster)  [unwired: 8 in, 1 out]
            n155 = call <vilib>:"Clear Errors.vi"("error in (no error)"=w510) -> ("error out"=w507:errorcluster)  [unwired: 5 in, 1 out]
            n156 = call <vilib>:"connect.vi"("PLC Type"=PLC_Type."S7 1200" ("PLC Type 2"), "error in (no error)"=w507, "IP address"=w504) -> ("error out"=w509:errorcluster, "S7 Connection out"=w508:T4)  [unwired: 7 in]
          }
        }
        n157 = Unbundle By Name(w498) -> ("status"=w501:bool)
        n158 = Not(x=w501) -> (.not. x?=w500:bool)
        "PLC 4" <- w500
        n159 = global write "Global 1.vi" "PLC 4"(w500) -> ()
      }
    }
    n160 = call "PADMINI_STOP_ALL.vi"("Enum"=enum16{"Read", "Write"}."Read") -> ("Boolean 2"=w413:bool)  [unwired: 9 in, 1 out]
    n161 = local read "stop"() -> (w412:bool)
    n162 = Or(x=w412, y=w413) -> (x .or. y?=w411:bool)
    n163 = Wait (ms)(milliseconds to wait=u32 50) -> ()  [unwired: 1 out]
  }
  n164 = while {
    shift-right: [w515] -> w107
    shift-left: w13 -> [w525]
    shift-right: [w523] -> w108
    shift-left: w14 -> [w524]
    tunnel: w106 -> [w514]
    stop <- w517 stop-if-true
    # "OP 60"
    n165 = flat-sequence {
      tunnel: [w534] -> w521
      tunnel: [w556] -> w516
      tunnel: w524 -> [w575]
      tunnel: w525 -> [w574]
      tunnel: w514 -> [w555]
      tunnel: [w555] -> w513
      tunnel: [w603] -> w523
      tunnel: [w602] -> w515
      tunnel: w521 -> [w605]
      tunnel: w516 -> [w604]
      tunnel: w513 -> [w601]
      frame #0 {
        w551 = u16 44 ("Data Block #")
        w531 = u16 43 ("Data Block #")
        # "AUTO WRITE"
        n166 = global read "DATA LOG.vi" "OP 60 Outputs"() -> (w573:bool)
        n167 = case shown="True" w573 {
          tunnel: w574 -> [w586 w599]
          tunnel: [w587 w588] -> w543
          tunnel: [w586 w591] -> w542
          tunnel: w575 -> [w587 w596]
          frame False {
          }
          frame True {
            w600 = u16 44  # Data Block #
            n168 = call "PADMINI_AUTO_BARCODE_STATUS 60.vi"("Enum"=enum16{"Read", "Write"}."Read", "error in (no error)"=w596) -> ("error out"=w595:errorcluster, "O/P"=w597:i32[])  [unwired: 8 in]
            n169 = global write "DATA LOG.vi" "OP 60 Outputs"(FALSE) -> ()
            n170 = call-poly <vilib>:"write DB.vi"("DINT input array"=w597, "error in (no error)"=w595, "Data Block #"=w600, "S7 Connection in"=w599) -> ("error out"=w589:errorcluster, "S7 Connection out"=w590:T4)  [unwired: 4 in, 2 out]
            n171 = call-poly <vilib>:"write DB.vi"("DINT input array"=i32[] [0] ("Data Byte"), "error in (no error)"=w589, "Data Block #"=u16 43, "S7 Connection in"=w590) -> ("error out"=w588:errorcluster, "S7 Connection out"=w591:T4)  [unwired: 4 in, 2 out]
          }
        }
        n172 = global read "DATA LOG.vi" "OP 60 reset"() -> (w541:bool)
        n173 = global read "DATA LOG.vi" "Auto Cycle On"() -> (w528:bool)
        n174 = case shown="True" w541 {
          tunnel: w543 -> [w576 w585]
          tunnel: [w576 w584] -> w544
          tunnel: w542 -> [w577 w583]
          tunnel: [w577 w582] -> w545
          frame False {
          }
          frame True {
            n175 = global write "DATA LOG.vi" "OP 60 reset"(FALSE) -> ()
            n176 = call-poly <vilib>:"write DB.vi"("Item offset [byte]"=u16 4 ("Data Block #"), "DINT input array"=i32[] [0], "error in (no error)"=w585, "Data Block #"=u16 43, "S7 Connection in"=w583) -> ("error out"=w584:errorcluster, "S7 Connection out"=w582:T4)  [unwired: 3 in, 2 out]
          }
        }
        n177 = Boolean To (0,1)(Boolean=w528) -> (0, 1=w527:i16)
        n178 = Build Array(w527) -> (w526:i16[])
        n179 = global read "Global 1.vi" "Filtered BARCODE selected"() -> (w554:string[])
        n180 = call-poly <vilib>:"write DB.vi"("Item offset [byte]"=u32 20, "DINT input array"=w526, "error in (no error)"=w544, "Data Block #"=w551, "S7 Connection in"=w545) -> ("error out"=w549:errorcluster, "S7 Connection out"=w548:T4)  [unwired: 3 in, 2 out]
        n181 = call-poly <vilib>:"write DB.vi"("Item offset [byte]"=u32 24, "Input STRINGS"=w554, "error in (no error)"=w549, "String length reserved in DB (default=254)"=u16 15, "Data Block #"=w551, "S7 Connection in"=w548) -> ("error out"=w546:errorcluster, "S7 Connection out"=w547:T4)  [unwired: 2 in, 2 out]
        n182 = call-poly <vilib>:"read DB.vi"("error in (no error)"=w546, "items #"=u16 2 ("Items # [byte]"), "Data Block #"=w531, "S7 Connection in"=w547) -> ("error out"=w571:errorcluster, "DINT result array"=w569:i32[], "S7 Connection out"=w566:T4)  [unwired: 5 in]
        n183 = call "PADMINI_AUTO_CYCLE STATE 60.vi"("Enum"=enum16{"Read", "Write"}."Write", "error in (no error)"=w571, "Input"=w569) -> ("error out"=w567:errorcluster)  [unwired: 7 in, 1 out]
        n184 = call-poly <vilib>:"read DB.vi"("Item offset [byte]"=u32 8, "error in (no error)"=w567, "items #"=u16 6 ("Items # [byte]"), "Data Block #"=w531, "S7 Connection in"=w566) -> ("error out"=w559:errorcluster, "REAL result array"=w557:sgl[], "S7 Connection out"=w565:T4)  [unwired: 4 in]
        n185 = call "PADMINI_AUTO_CYCLE VALUE 60.vi"("Enum"=enum16{"Read", "Write"}."Write", "error in (no error)"=w559, "Input"=w557) -> ("error out"=w558:errorcluster)  [unwired: 7 in, 1 out]
        n186 = call-poly <vilib>:"read DB.vi"("Item offset [byte]"=u32 32, "String length reserved in DB (default=254)"=u16 50, "error in (no error)"=w558, "items #"=u16 1 ("Items # [byte]"), "Data Block #"=w531, "S7 Connection in"=w565) -> ("error out"=w536:errorcluster, "STRING result Array"=w533:string[], "S7 Connection out"=w535:T4)  [unwired: 2 in, 1 out]
        n187 = call-poly <vilib>:"read DB.vi"("Item offset [byte]"=u32 84, "String length reserved in DB (default=254)"=u16 10, "error in (no error)"=w536, "items #"=u16 7 ("Items # [byte]"), "Data Block #"=w531, "S7 Connection in"=w535) -> ("error out"=w537:errorcluster, "STRING result Array"=w540:string[], "S7 Connection out"=w534:T4)  [unwired: 2 in, 1 out]
        n188 = Build Array (concatenate)(w533, w540) -> (w532:string[])
        n189 = call "PADMINI_AUTO_BARCODE_STRING 60.vi"("Enum"=enum16{"Read", "Write"}."Write", "error in (no error)"=w537, "Input"=w532) -> ("error out"=w556:errorcluster)  [unwired: 7 in, 1 out]
      }
      frame #1 {
        # "RECONNECT"
        n190 = case shown="Error" w604 {
          selector: w604 -> [w609 w617]
          tunnel: [w608 w614] -> w602
          tunnel: [w609 w615] -> w603
          tunnel: w605 -> [w608 w611]
          tunnel: w601 -> [_ w610]
          frame No Error {
          }
          frame Error {
            n191 = call <vilib>:"Clear Errors.vi"("error in (no error)"=w617) -> ("error out"=w618:errorcluster)  [unwired: 5 in, 1 out]
            n192 = call <vilib>:"disconnect.vi"("error in (no error)"=w618, "S7 Connection in"=w611) -> ("error out"=w616:errorcluster)  [unwired: 8 in, 1 out]
            n193 = call <vilib>:"Clear Errors.vi"("error in (no error)"=w616) -> ("error out"=w613:errorcluster)  [unwired: 5 in, 1 out]
            n194 = call <vilib>:"connect.vi"("PLC Type"=PLC_Type."S7 1200" ("PLC Type 2"), "error in (no error)"=w613, "IP address"=w610) -> ("error out"=w615:errorcluster, "S7 Connection out"=w614:T4)  [unwired: 7 in]
          }
        }
        n195 = Unbundle By Name(w604) -> ("status"=w607:bool)
        n196 = Not(x=w607) -> (.not. x?=w606:bool)
        "PLC 5" <- w606
        n197 = global write "Global 1.vi" "PLC 5"(w606) -> ()
      }
    }
    n198 = call "PADMINI_STOP_ALL.vi"("Enum"=enum16{"Read", "Write"}."Read") -> ("Boolean 2"=w519:bool)  [unwired: 9 in, 1 out]
    n199 = local read "stop"() -> (w518:bool)
    n200 = Or(x=w518, y=w519) -> (x .or. y?=w517:bool)
    n201 = Wait (ms)(milliseconds to wait=u32 50) -> ()  [unwired: 1 out]
  }
  n202 = while {
    shift-right: [w621] -> w89
    shift-left: w8 -> [w631]
    shift-right: [w629] -> w90
    shift-left: w9 -> [w630]
    tunnel: w66 -> [w620]
    stop <- w623 stop-if-true
    # "OP 70 - 80"
    n203 = flat-sequence {
      tunnel: [w642] -> w627
      tunnel: [w690] -> w622
      tunnel: w630 -> [w728]
      tunnel: w631 -> [w727]
      tunnel: w620 -> [w709]
      tunnel: [w709] -> w619
      tunnel: [w781] -> w629
      tunnel: [w780] -> w621
      tunnel: w627 -> [w783]
      tunnel: w622 -> [w782]
      tunnel: w619 -> [w779]
      frame #0 {
        w658 = u16 83 ("Data Block #")
        w683 = u16 81 ("Data Block #")
        w641 = u16 82 ("Data Block #")
        w664 = u16 80 ("Data Block #")
        # "AUTO WRITE"
        n204 = global read "DATA LOG.vi" "OP 70 Outputs"() -> (w726:bool)
        n205 = case shown="True" w726 {
          tunnel: w727 -> [w764 w777]
          tunnel: [w765 w768] -> w688
          tunnel: [w764 w769] -> w687
          tunnel: w728 -> [w765 w774]
          frame False {
          }
          frame True {
            w778 = u16 81  # Data Block #
            n206 = call "PADMINI_AUTO_BARCODE_STATUS 70.vi"("Enum"=enum16{"Read", "Write"}."Read", "error in (no error)"=w774) -> ("error out"=w773:errorcluster, "O/P"=w775:i32[])  [unwired: 8 in]
            n207 = global write "DATA LOG.vi" "OP 70 Outputs"(FALSE) -> ()
            n208 = call-poly <vilib>:"write DB.vi"("DINT input array"=w775, "error in (no error)"=w773, "Data Block #"=w778, "S7 Connection in"=w777) -> ("error out"=w766:errorcluster, "S7 Connection out"=w767:T4)  [unwired: 4 in, 2 out]
            n209 = call-poly <vilib>:"write DB.vi"("DINT input array"=i32[] [0] ("Data Byte"), "error in (no error)"=w766, "Data Block #"=u16 80, "S7 Connection in"=w767) -> ("error out"=w768:errorcluster, "S7 Connection out"=w769:T4)  [unwired: 4 in, 2 out]
          }
        }
        n210 = global read "DATA LOG.vi" "OP 70 reset"() -> (w689:bool)
        n211 = global read "DATA LOG.vi" "Auto Cycle On"() -> (w634:bool)
        n212 = case shown="True" w689 {
          tunnel: w688 -> [w739 w748]
          tunnel: [w739 w747] -> w678
          tunnel: w687 -> [w740 w746]
          tunnel: [w740 w745] -> w679
          frame False {
          }
          frame True {
            n213 = global write "DATA LOG.vi" "OP 70 reset"(FALSE) -> ()
            n214 = call-poly <vilib>:"write DB.vi"("Item offset [byte]"=u16 4 ("Data Block #"), "DINT input array"=i32[] [0], "error in (no error)"=w748, "Data Block #"=u16 80, "S7 Connection in"=w746) -> ("error out"=w747:errorcluster, "S7 Connection out"=w745:T4)  [unwired: 3 in, 2 out]
          }
        }
        n215 = Boolean To (0,1)(Boolean=w634) -> (0, 1=w633:i16)
        n216 = Build Array(w633) -> (w632:i16[])
        n217 = global read "Global 1.vi" "Filtered BARCODE selected"() -> (w680:string[])
        n218 = call-poly <vilib>:"write DB.vi"("Item offset [byte]"=u32 20, "DINT input array"=w632, "error in (no error)"=w678, "Data Block #"=w683, "S7 Connection in"=w679) -> ("error out"=w685:errorcluster, "S7 Connection out"=w686:T4)  [unwired: 3 in, 2 out]
        n219 = call-poly <vilib>:"write DB.vi"("Item offset [byte]"=u32 24, "Input STRINGS"=w680, "error in (no error)"=w685, "String length reserved in DB (default=254)"=u16 15, "Data Block #"=w683, "S7 Connection in"=w686) -> ("error out"=w676:errorcluster, "S7 Connection out"=w677:T4)  [unwired: 2 in, 2 out]
        n220 = call-poly <vilib>:"read DB.vi"("error in (no error)"=w676, "items #"=u16 2 ("Items # [byte]"), "Data Block #"=w664, "S7 Connection in"=w677) -> ("error out"=w724:errorcluster, "DINT result array"=w722:i32[], "S7 Connection out"=w719:T4)  [unwired: 5 in]
        n221 = call "PADMINI_AUTO_CYCLE STATE 70.vi"("Enum"=enum16{"Read", "Write"}."Write", "error in (no error)"=w724, "Input"=w722) -> ("error out"=w720:errorcluster)  [unwired: 7 in, 1 out]
        n222 = call-poly <vilib>:"read DB.vi"("Item offset [byte]"=u32 8, "error in (no error)"=w720, "items #"=u16 2 ("Items # [byte]"), "Data Block #"=w664, "S7 Connection in"=w719) -> ("error out"=w712:errorcluster, "REAL result array"=w710:sgl[], "S7 Connection out"=w718:T4)  [unwired: 4 in]
        n223 = call "PADMINI_AUTO_CYCLE VALUE 70.vi"("Enum"=enum16{"Read", "Write"}."Write", "error in (no error)"=w712, "Input"=w710) -> ("error out"=w711:errorcluster)  [unwired: 7 in, 1 out]
        n224 = call-poly <vilib>:"read DB.vi"("Item offset [byte]"=u32 16, "String length reserved in DB (default=254)"=u16 50, "error in (no error)"=w711, "items #"=u16 1 ("Items # [byte]"), "Data Block #"=w664, "S7 Connection in"=w718) -> ("error out"=w669:errorcluster, "STRING result Array"=w668:string[], "S7 Connection out"=w670:T4)  [unwired: 2 in, 1 out]
        n225 = call-poly <vilib>:"read DB.vi"("Item offset [byte]"=u32 68, "String length reserved in DB (default=254)"=u16 10, "error in (no error)"=w669, "items #"=u16 1 ("Items # [byte]"), "Data Block #"=w664, "S7 Connection in"=w670) -> ("error out"=w671:errorcluster, "STRING result Array"=w672:string[], "S7 Connection out"=w665:T4)  [unwired: 2 in, 1 out]
        n226 = Build Array (concatenate)(w668, w672) -> (w666:string[])
        n227 = call "PADMINI_AUTO_BARCODE_STRING 70.vi"("Enum"=enum16{"Read", "Write"}."Write", "error in (no error)"=w671, "Input"=w666) -> ("error out"=w691:errorcluster)  [unwired: 7 in, 1 out]
        n228 = global read "DATA LOG.vi" "OP 80 Outputs"() -> (w692:bool)
        n229 = case shown="True" w692 {
          tunnel: [w750 w753] -> w663
          tunnel: [w749 w754] -> w639
          tunnel: w691 -> [w750 w760]
          tunnel: w665 -> [w749 w757]
          frame False {
          }
          frame True {
            w763 = u16 83  # Data Block #
            n230 = call "PADMINI_AUTO_BARCODE_STATUS 80.vi"("Enum"=enum16{"Read", "Write"}."Read", "error in (no error)"=w760) -> ("error out"=w759:errorcluster, "O/P"=w761:i32[])  [unwired: 8 in]
            n231 = global write "DATA LOG.vi" "OP 80 Outputs"(FALSE) -> ()
            n232 = call-poly <vilib>:"write DB.vi"("DINT input array"=w761, "error in (no error)"=w759, "Data Block #"=w763, "S7 Connection in"=w757) -> ("error out"=w751:errorcluster, "S7 Connection out"=w752:T4)  [unwired: 4 in, 2 out]
            n233 = call-poly <vilib>:"write DB.vi"("DINT input array"=i32[] [0] ("Data Byte"), "error in (no error)"=w751, "Data Block #"=u16 82, "S7 Connection in"=w752) -> ("error out"=w753:errorcluster, "S7 Connection out"=w754:T4)  [unwired: 4 in, 2 out]
          }
        }
        n234 = global read "DATA LOG.vi" "OP 80 reset"() -> (w662:bool)
        n235 = global read "DATA LOG.vi" "Auto Cycle On"() -> (w637:bool)
        n236 = case shown="True" w662 {
          tunnel: w663 -> [w730 w738]
          tunnel: [w730 w733] -> _
          tunnel: [w730 w733] -> w652
          tunnel: w639 -> [w729 w732]
          tunnel: [w729 w731] -> w638
          frame False {
          }
          frame True {
            n237 = global write "DATA LOG.vi" "OP 80 reset"(FALSE) -> ()
            n238 = call-poly <vilib>:"write DB.vi"("Item offset [byte]"=u16 4 ("Data Block #"), "DINT input array"=i32[] [0], "error in (no error)"=w738, "Data Block #"=u16 82, "S7 Connection in"=w732) -> ("error out"=w733:errorcluster, "S7 Connection out"=w731:T4)  [unwired: 3 in, 2 out]
          }
        }
        n239 = Boolean To (0,1)(Boolean=w637) -> (0, 1=w636:i16)
        n240 = Build Array(w636) -> (w635:i16[])
        n241 = global read "Global 1.vi" "Filtered BARCODE selected"() -> (w655:string[])
        n242 = call-poly <vilib>:"write DB.vi"("Item offset [byte]"=u32 20, "DINT input array"=w635, "error in (no error)"=w652, "Data Block #"=w658, "S7 Connection in"=w638) -> ("error out"=w660:errorcluster, "S7 Connection out"=w661:T4)  [unwired: 3 in, 2 out]
        n243 = call-poly <vilib>:"write DB.vi"("Item offset [byte]"=u32 24, "Input STRINGS"=w655, "error in (no error)"=w660, "String length reserved in DB (default=254)"=u16 15, "Data Block #"=w658, "S7 Connection in"=w661) -> ("error out"=w653:errorcluster, "S7 Connection out"=w654:T4)  [unwired: 2 in, 2 out]
        n244 = call-poly <vilib>:"read DB.vi"("error in (no error)"=w653, "items #"=u16 2 ("Items # [byte]"), "Data Block #"=w641, "S7 Connection in"=w654) -> ("error out"=w694:errorcluster, "DINT result array"=w696:i32[], "S7 Connection out"=w699:T4)  [unwired: 5 in]
        n245 = call "PADMINI_AUTO_CYCLE STATE 80.vi"("Enum"=enum16{"Read", "Write"}."Write", "error in (no error)"=w694, "Input"=w696) -> ("error out"=w698:errorcluster)  [unwired: 7 in, 1 out]
        n246 = call-poly <vilib>:"read DB.vi"("Item offset [byte]"=u32 8, "error in (no error)"=w698, "items #"=u16 1 ("Items # [byte]"), "Data Block #"=w641, "S7 Connection in"=w699) -> ("error out"=w706:errorcluster, "REAL result array"=w708:sgl[], "S7 Connection out"=w700:T4)  [unwired: 4 in]
        n247 = call "PADMINI_AUTO_CYCLE VALUE 80.vi"("Enum"=enum16{"Read", "Write"}."Write", "error in (no error)"=w706, "Input"=w708) -> ("error out"=w707:errorcluster)  [unwired: 7 in, 1 out]
        n248 = call-poly <vilib>:"read DB.vi"("Item offset [byte]"=u32 12, "String length reserved in DB (default=254)"=u16 50, "error in (no error)"=w707, "items #"=u16 1 ("Items # [byte]"), "Data Block #"=w641, "S7 Connection in"=w700) -> ("error out"=w647:errorcluster, "STRING result Array"=w645:string[], "S7 Connection out"=w643:T4)  [unwired: 2 in, 1 out]
        n249 = call-poly <vilib>:"read DB.vi"("Item offset [byte]"=u32 64, "String length reserved in DB (default=254)"=u16 10, "error in (no error)"=w647, "items #"=u16 2 ("Items # [byte]"), "Data Block #"=w641, "S7 Connection in"=w643) -> ("error out"=w646:errorcluster, "STRING result Array"=w651:string[], "S7 Connection out"=w642:T4)  [unwired: 2 in, 1 out]
        n250 = Build Array (concatenate)(w645, w651) -> (w644:string[])
        n251 = call "PADMINI_AUTO_BARCODE_STRING 80.vi"("Enum"=enum16{"Read", "Write"}."Write", "error in (no error)"=w646, "Input"=w644) -> ("error out"=w690:errorcluster)  [unwired: 7 in, 1 out]
      }
      frame #1 {
        # "RECONNECT"
        n252 = case shown="Error" w782 {
          selector: w782 -> [w787 w795]
          tunnel: [w786 w792] -> w780
          tunnel: [w787 w793] -> w781
          tunnel: w783 -> [w786 w789]
          tunnel: w779 -> [_ w788]
          frame No Error {
          }
          frame Error {
            n253 = call <vilib>:"Clear Errors.vi"("error in (no error)"=w795) -> ("error out"=w796:errorcluster)  [unwired: 5 in, 1 out]
            n254 = call <vilib>:"disconnect.vi"("error in (no error)"=w796, "S7 Connection in"=w789) -> ("error out"=w794:errorcluster)  [unwired: 8 in, 1 out]
            n255 = call <vilib>:"Clear Errors.vi"("error in (no error)"=w794) -> ("error out"=w791:errorcluster)  [unwired: 5 in, 1 out]
            n256 = call <vilib>:"connect.vi"("PLC Type"=PLC_Type."S7 1200" ("PLC Type 2"), "error in (no error)"=w791, "IP address"=w788) -> ("error out"=w793:errorcluster, "S7 Connection out"=w792:T4)  [unwired: 7 in]
          }
        }
        n257 = Unbundle By Name(w782) -> ("status"=w785:bool)
        n258 = Not(x=w785) -> (.not. x?=w784:bool)
        "PLC 6" <- w784
        n259 = global write "Global 1.vi" "PLC 6"(w784) -> ()
      }
    }
    n260 = call "PADMINI_STOP_ALL.vi"("Enum"=enum16{"Read", "Write"}."Read") -> ("Boolean 2"=w625:bool)  [unwired: 9 in, 1 out]
    n261 = local read "stop"() -> (w624:bool)
    n262 = Or(x=w624, y=w625) -> (x .or. y?=w623:bool)
    n263 = Wait (ms)(milliseconds to wait=u32 50) -> ()  [unwired: 1 out]
  }
  n264 = while {
    shift-right: [w799] -> w61
    shift-left: w4 -> [w809]
    shift-right: [w807] -> w62
    shift-left: w3 -> [w808]
    tunnel: w65 -> [w798]
    stop <- w801 stop-if-true
    # "OP 90 - 100 - 110"
    n265 = flat-sequence {
      tunnel: [w885] -> w805
      tunnel: [w886] -> w800
      tunnel: w808 -> [w924]
      tunnel: w809 -> [w923]
      tunnel: w798 -> [w905]
      tunnel: [w905] -> w797
      tunnel: [w992] -> w807
      tunnel: [w991] -> w799
      tunnel: w805 -> [w994]
      tunnel: w800 -> [w993]
      tunnel: w797 -> [w990]
      frame #0 {
        w826 = u16 75 ("Data Block #")
        w851 = u16 72 ("Data Block #")
        w877 = u16 70 ("Data Block #")
        w835 = u16 71 ("Data Block #")
        w865 = u16 69 ("Data Block #")
        # "OP100 OK\nOP 100 NG"
        # "AUTO WRITE"
        n266 = global read "DATA LOG.vi" "OP 90 Outputs"() -> (w922:bool)
        n267 = case shown="True" w922 {
          tunnel: w923 -> [w975 w988]
          tunnel: [w976 w977] -> w882
          tunnel: [w975 w978] -> w883
          tunnel: w924 -> [w976 w985]
          frame False {
          }
          frame True {
            w989 = u16 70  # Data Block #
            n268 = call "PADMINI_AUTO_BARCODE_STATUS 90.vi"("Enum"=enum16{"Read", "Write"}."Read", "error in (no error)"=w985) -> ("error out"=w984:errorcluster, "O/P"=w986:i32[])  [unwired: 8 in]
            n269 = global write "DATA LOG.vi" "OP 90 Outputs"(FALSE) -> ()
            n270 = call-poly <vilib>:"write DB.vi"("DINT input array"=w986, "error in (no error)"=w984, "Data Block #"=w989, "S7 Connection in"=w988) -> ("error out"=w980:errorcluster, "S7 Connection out"=w979:T4)  [unwired: 4 in, 2 out]
            n271 = call-poly <vilib>:"write DB.vi"("DINT input array"=i32[] [0] ("Data Byte"), "error in (no error)"=w980, "Data Block #"=u16 69, "S7 Connection in"=w979) -> ("error out"=w977:errorcluster, "S7 Connection out"=w978:T4)  [unwired: 4 in, 2 out]
          }
        }
        n272 = global read "DATA LOG.vi" "OP 90 reset"() -> (w881:bool)
        n273 = case shown="True" w881 {
          tunnel: w882 -> [w950 w959]
          tunnel: [w950 w958] -> w870
          tunnel: w883 -> [w951 w957]
          tunnel: [w951 w956] -> w871
          frame False {
          }
          frame True {
            n274 = global write "DATA LOG.vi" "OP 90 reset"(FALSE) -> ()
            n275 = call-poly <vilib>:"write DB.vi"("Item offset [byte]"=u16 4 ("Data Block #"), "DINT input array"=i32[] [0], "error in (no error)"=w959, "Data Block #"=u16 69, "S7 Connection in"=w957) -> ("error out"=w958:errorcluster, "S7 Connection out"=w956:T4)  [unwired: 3 in, 2 out]
          }
        }
        n276 = global read "DATA LOG.vi" "Auto Cycle On"() -> (w817:bool)
        n277 = Boolean To (0,1)(Boolean=w817) -> (0, 1=w816:i16)
        n278 = Build Array(w816) -> (w815:i16[])
        n279 = global read "Global 1.vi" "Filtered BARCODE selected"() -> (w880:string[])
        n280 = call-poly <vilib>:"write DB.vi"("Item offset [byte]"=u32 20, "DINT input array"=w815, "error in (no error)"=w870, "Data Block #"=w877, "S7 Connection in"=w871) -> ("error out"=w875:errorcluster, "S7 Connection out"=w874:T4)  [unwired: 3 in, 2 out]
        n281 = call-poly <vilib>:"write DB.vi"("Item offset [byte]"=u32 24, "Input STRINGS"=w880, "error in (no error)"=w875, "String length reserved in DB (default=254)"=u16 15, "Data Block #"=w877, "S7 Connection in"=w874) -> ("error out"=w872:errorcluster, "S7 Connection out"=w873:T4)  [unwired: 2 in, 2 out]
        n282 = call-poly <vilib>:"read DB.vi"("error in (no error)"=w872, "items #"=u16 2 ("Items # [byte]"), "Data Block #"=w865, "S7 Connection in"=w873) -> ("error out"=w920:errorcluster, "DINT result array"=w918:i32[], "S7 Connection out"=w915:T4)  [unwired: 5 in]
        n283 = call "PADMINI_AUTO_CYCLE STATE 90.vi"("Enum"=enum16{"Read", "Write"}."Write", "error in (no error)"=w920, "Input"=w918) -> ("error out"=w916:errorcluster)  [unwired: 7 in, 1 out]
        n284 = call-poly <vilib>:"read DB.vi"("Item offset [byte]"=u32 8, "error in (no error)"=w916, "items #"=u16 2 ("Items # [byte]"), "Data Block #"=w865, "S7 Connection in"=w915) -> ("error out"=w908:errorcluster, "REAL result array"=w906:sgl[], "S7 Connection out"=w914:T4)  [unwired: 4 in]
        n285 = call "PADMINI_AUTO_CYCLE VALUE 90.vi"("Enum"=enum16{"Read", "Write"}."Write", "error in (no error)"=w908, "Input"=w906) -> ("error out"=w907:errorcluster)  [unwired: 7 in, 1 out]
        n286 = call-poly <vilib>:"read DB.vi"("Item offset [byte]"=u32 16, "String length reserved in DB (default=254)"=u16 50, "error in (no error)"=w907, "items #"=u16 1 ("Items # [byte]"), "Data Block #"=w865, "S7 Connection in"=w914) -> ("error out"=w869:errorcluster, "STRING result Array"=w860:string[], "S7 Connection out"=w868:T4)  [unwired: 2 in, 1 out]
        n287 = call-poly <vilib>:"read DB.vi"("Item offset [byte]"=u32 68, "String length reserved in DB (default=254)"=u16 10, "error in (no error)"=w869, "items #"=u16 3 ("Items # [byte]"), "Data Block #"=w865, "S7 Connection in"=w868) -> ("error out"=w867:errorcluster, "STRING result Array"=w859:string[], "S7 Connection out"=w866:T4)  [unwired: 2 in, 1 out]
        n288 = Build Array (concatenate)(w860, w859) -> (w858:string[])
        n289 = call "PADMINI_AUTO_BARCODE_STRING 90.vi"("Enum"=enum16{"Read", "Write"}."Write", "error in (no error)"=w867, "Input"=w858) -> ("error out"=w887:errorcluster)  [unwired: 7 in, 1 out]
        n290 = global read "DATA LOG.vi" "OP 100 Outputs"() -> (w888:bool)
        n291 = case shown="True" w888 {
          tunnel: w866 -> [w960 w973]
          tunnel: [w961 w964] -> w856
          tunnel: [w960 w965] -> w857
          tunnel: w887 -> [w961 w970]
          frame False {
          }
          frame True {
            w974 = u16 72  # Data Block #
            n292 = call "PADMINI_AUTO_BARCODE_STATUS 100.vi"("Enum"=enum16{"Read", "Write"}."Read", "error in (no error)"=w970) -> ("error out"=w969:errorcluster, "O/P"=w971:i32[])  [unwired: 8 in]
            n293 = global write "DATA LOG.vi" "OP 100 Outputs"(FALSE) -> ()
            n294 = call-poly <vilib>:"write DB.vi"("DINT input array"=w971, "error in (no error)"=w969, "Data Block #"=w974, "S7 Connection in"=w973) -> ("error out"=w963:errorcluster, "S7 Connection out"=w962:T4)  [unwired: 4 in, 2 out]
            n295 = call-poly <vilib>:"write DB.vi"("DINT input array"=i32[] [0] ("Data Byte"), "error in (no error)"=w963, "Data Block #"=u16 71, "S7 Connection in"=w962) -> ("error out"=w964:errorcluster, "S7 Connection out"=w965:T4)  [unwired: 4 in, 2 out]
          }
        }
        n296 = global read "DATA LOG.vi" "OP 100 reset"() -> (w855:bool)
        n297 = case shown="True" w855 {
          tunnel: w856 -> [w940 w949]
          tunnel: [w940 w948] -> w847
          tunnel: w857 -> [w941 w947]
          tunnel: [w941 w946] -> w846
          frame False {
          }
          frame True {
            n298 = global write "DATA LOG.vi" "OP 100 reset"(FALSE) -> ()
            n299 = call-poly <vilib>:"write DB.vi"("Item offset [byte]"=u16 4 ("Data Block #"), "DINT input array"=i32[] [0], "error in (no error)"=w949, "Data Block #"=u16 71, "S7 Connection in"=w947) -> ("error out"=w948:errorcluster, "S7 Connection out"=w946:T4)  [unwired: 3 in, 2 out]
          }
        }
        n300 = global read "DATA LOG.vi" "Auto Cycle On"() -> (w814:bool)
        n301 = Boolean To (0,1)(Boolean=w814) -> (0, 1=w813:i16)
        n302 = Build Array(w813) -> (w812:i16[])
        n303 = global read "Global 1.vi" "Filtered BARCODE selected"() -> (w848:string[])
        n304 = call-poly <vilib>:"write DB.vi"("Item offset [byte]"=u32 20, "DINT input array"=w812, "error in (no error)"=w847, "Data Block #"=w851, "S7 Connection in"=w846) -> ("error out"=w853:errorcluster, "S7 Connection out"=w854:T4)  [unwired: 3 in, 2 out]
        n305 = call-poly <vilib>:"write DB.vi"("Item offset [byte]"=u32 24, "Input STRINGS"=w848, "error in (no error)"=w853, "String length reserved in DB (default=254)"=u16 15, "Data Block #"=w851, "S7 Connection in"=w854) -> ("error out"=w844:errorcluster, "S7 Connection out"=w845:T4)  [unwired: 2 in, 2 out]
        n306 = call-poly <vilib>:"read DB.vi"("error in (no error)"=w844, "items #"=u16 2 ("Items # [byte]"), "Data Block #"=w835, "S7 Connection in"=w845) -> ("error out"=w890:errorcluster, "DINT result array"=w892:i32[], "S7 Connection out"=w895:T4)  [unwired: 5 in]
        n307 = call "PADMINI_AUTO_CYCLE STATE 100.vi"("Enum"=enum16{"Read", "Write"}."Write", "error in (no error)"=w890, "Input"=w892) -> ("error out"=w894:errorcluster)  [unwired: 7 in, 1 out]
        n308 = call-poly <vilib>:"read DB.vi"("Item offset [byte]"=u32 8, "error in (no error)"=w894, "items #"=u16 11 ("Items # [byte]"), "Data Block #"=w835, "S7 Connection in"=w895) -> ("error out"=w902:errorcluster, "REAL result array"=w904:sgl[], "S7 Connection out"=w896:T4)  [unwired: 4 in]
        n309 = call "PADMINI_AUTO_CYCLE VALUE 100.vi"("Enum"=enum16{"Read", "Write"}."Write", "error in (no error)"=w902, "Input"=w904) -> ("error out"=w903:errorcluster)  [unwired: 7 in, 1 out]
        n310 = call-poly <vilib>:"read DB.vi"("Item offset [byte]"=u32 52, "String length reserved in DB (default=254)"=u16 50, "error in (no error)"=w903, "items #"=u16 1 ("Items # [byte]"), "Data Block #"=w835, "S7 Connection in"=w896) -> ("error out"=w841:errorcluster, "STRING result Array"=w838:string[], "S7 Connection out"=w840:T4)  [unwired: 2 in, 1 out]
        n311 = call-poly <vilib>:"read DB.vi"("Item offset [byte]"=u32 104, "String length reserved in DB (default=254)"=u16 10, "error in (no error)"=w841, "items #"=u16 2 ("Items # [byte]"), "Data Block #"=w835, "S7 Connection in"=w840) -> ("error out"=w842:errorcluster, "STRING result Array"=w836:string[], "S7 Connection out"=w839:T4)  [unwired: 2 in, 1 out]
        n312 = Build Array (concatenate)(w838, w836) -> (w837:string[])
        n313 = call "PADMINI_AUTO_BARCODE_STRING 100.vi"("Enum"=enum16{"Read", "Write"}."Write", "error in (no error)"=w842, "Input"=w837) -> ("error out"=w884:errorcluster)  [unwired: 7 in, 1 out]
        n314 = global read "DATA LOG.vi" "OP 110 Outputs"() -> (w832:bool)
        n315 = case shown="True" w832 {
          tunnel: [w925 w930] -> w818
          tunnel: [w926 w931] -> w819
          tunnel: w884 -> [w925 w935]
          tunnel: w839 -> [w926 w934]
          frame False {
          }
          frame True {
            w927 = i32[] [0]  # DINT input array
            w928 = u16 75  # Data Block #
            n316 = call "PADMINI_AUTO_BARCODE_STATUS 110.vi"("Enum"=enum16{"Read", "Write"}."Read", "error in (no error)"=w935) -> ("error out"=w937:errorcluster, "O/P"=w938:i32[])  [unwired: 8 in]
            n317 = call-poly <vilib>:"write DB.vi"("Item offset [byte]"=u32 4, "DINT input array"=w938, "error in (no error)"=w937, "Data Block #"=w928, "S7 Connection in"=w934) -> ("error out"=w929:errorcluster, "S7 Connection out"=w932:T4)  [unwired: 3 in, 2 out]
            n318 = global write "DATA LOG.vi" "OP 110 Outputs"(FALSE) -> ()
            n319 = call-poly <vilib>:"write DB.vi"("DINT input array"=w927, "error in (no error)"=w929, "Data Block #"=w928, "S7 Connection in"=w932) -> ("error out"=w930:errorcluster, "S7 Connection out"=w931:T4)  [unwired: 4 in, 2 out]
          }
        }
        n320 = call-poly <vilib>:"read DB.vi"("error in (no error)"=w818, "items #"=u16 1 ("Items # [byte]"), "Data Block #"=w826, "S7 Connection in"=w819) -> ("error out"=w830:errorcluster, "DINT result array"=w828:i32[], "S7 Connection out"=w827:T4)  [unwired: 5 in]
        n321 = call "PADMINI_AUTO_CYCLE STATE 110.vi"("Enum"=enum16{"Read", "Write"}."Write", "error in (no error)"=w830, "Input"=w828) -> ("error out"=w820:errorcluster)  [unwired: 7 in, 1 out]
        n322 = call-poly <vilib>:"read DB.vi"("Item offset [byte]"=u32 12, "String length reserved in DB (default=254)"=u16 50, "error in (no error)"=w820, "items #"=u16 1 ("Items # [byte]"), "Data Block #"=w826, "S7 Connection in"=w827) -> ("error out"=w822:errorcluster, "STRING result Array"=w823:string[], "S7 Connection out"=w885:T4)  [unwired: 2 in, 1 out]
        n323 = call "PADMINI_AUTO_BARCODE_STRING 110.vi"("Enum"=enum16{"Read", "Write"}."Write", "error in (no error)"=w822, "Input"=w823) -> ("error out"=w886:errorcluster)  [unwired: 7 in, 1 out]
      }
      frame #1 {
        # "RECONNECT"
        n324 = case shown="Error" w993 {
          selector: w993 -> [w998 w1006]
          tunnel: [w997 w1003] -> w991
          tunnel: [w998 w1004] -> w992
          tunnel: w994 -> [w997 w1000]
          tunnel: w990 -> [_ w999]
          frame No Error {
          }
          frame Error {
            n325 = call <vilib>:"Clear Errors.vi"("error in (no error)"=w1006) -> ("error out"=w1007:errorcluster)  [unwired: 5 in, 1 out]
            n326 = call <vilib>:"disconnect.vi"("error in (no error)"=w1007, "S7 Connection in"=w1000) -> ("error out"=w1005:errorcluster)  [unwired: 8 in, 1 out]
            n327 = call <vilib>:"Clear Errors.vi"("error in (no error)"=w1005) -> ("error out"=w1002:errorcluster)  [unwired: 5 in, 1 out]
            n328 = call <vilib>:"connect.vi"("PLC Type"=PLC_Type."S7 1200" ("PLC Type 2"), "error in (no error)"=w1002, "IP address"=w999) -> ("error out"=w1004:errorcluster, "S7 Connection out"=w1003:T4)  [unwired: 7 in]
          }
        }
        n329 = Unbundle By Name(w993) -> ("status"=w996:bool)
        n330 = Not(x=w996) -> (.not. x?=w995:bool)
        "PLC 7" <- w995
        n331 = global write "Global 1.vi" "PLC 7"(w995) -> ()
      }
    }
    n332 = call "PADMINI_STOP_ALL.vi"("Enum"=enum16{"Read", "Write"}."Read") -> ("Boolean 2"=w803:bool)  [unwired: 9 in, 1 out]
    n333 = local read "stop"() -> (w802:bool)
    n334 = Or(x=w802, y=w803) -> (x .or. y?=w801:bool)
    n335 = Wait (ms)(milliseconds to wait=u32 50) -> ()  [unwired: 1 out]
  }
  n336 = call <vilib>:"Clear Errors.vi"("error in (no error)"=w139) -> ("error out"=w140:errorcluster)  [unwired: 5 in, 1 out]
  n337 = call <vilib>:"Clear Errors.vi"("error in (no error)"=w146) -> ("error out"=w148:errorcluster)  [unwired: 5 in, 1 out]
  n338 = call <vilib>:"Clear Errors.vi"("error in (no error)"=w108) -> ("error out"=w109:errorcluster)  [unwired: 5 in, 1 out]
  n339 = call <vilib>:"Clear Errors.vi"("error in (no error)"=w125) -> ("error out"=w124:errorcluster)  [unwired: 5 in, 1 out]
  n340 = call <vilib>:"disconnect.vi"("error in (no error)"=w109, "S7 Connection in"=w107) -> ("error out"=w104:errorcluster)  [unwired: 8 in, 1 out]
  n341 = call <vilib>:"Clear Errors.vi"("error in (no error)"=w90) -> ("error out"=w91:errorcluster)  [unwired: 5 in, 1 out]
  n342 = call <vilib>:"disconnect.vi"("error in (no error)"=w91, "S7 Connection in"=w89) -> ("error out"=w60:errorcluster)  [unwired: 8 in, 1 out]
  n343 = call <vilib>:"disconnect.vi"("error in (no error)"=w124, "S7 Connection in"=w126) -> ("error out"=w105:errorcluster)  [unwired: 8 in, 1 out]
  n344 = call <vilib>:"disconnect.vi"("error in (no error)"=w148, "S7 Connection in"=w147) -> ("error out"=w136:errorcluster)  [unwired: 8 in, 1 out]
  n345 = call <vilib>:"disconnect.vi"("error in (no error)"=w140, "S7 Connection in"=w138) -> ("error out"=w137:errorcluster)  [unwired: 8 in, 1 out]
  n346 = call <vilib>:"Clear Errors.vi"("error in (no error)"=w62) -> ("error out"=w63:errorcluster)  [unwired: 5 in, 1 out]
  n347 = Merge Errors(w136, w137, w105, w104) -> (w135:errorcluster)
  n348 = call <vilib>:"Clear Errors.vi"("error in (no error)"=w185) -> ("error out"=w173:errorcluster)  [unwired: 5 in, 1 out]
  n349 = call <vilib>:"disconnect.vi"("error in (no error)"=w63, "S7 Connection in"=w61) -> ("error out"=w58:errorcluster)  [unwired: 8 in, 1 out]
  n350 = call <vilib>:"disconnect.vi"("error in (no error)"=w173, "S7 Connection in"=w172) -> ("error out"=w171:errorcluster)  [unwired: 8 in, 1 out]
  n351 = Merge Errors(w60, w58) -> (w59:errorcluster)
  n352 = Merge Errors(w171, w135, w59) -> (w190:errorcluster)
  n353 = call <vilib>:"Simple Error Handler.vi"("type of dialog (OK msg:1)"=w40, "error in (no error)"=w190) -> ("error out"=w189:errorcluster)  [unwired: 3 in, 4 out]
  n354 = control-ref of="This VI"() -> (w41:refnum<vi>)
  n355 = call <vilib>:"Clear Errors.vi"("error in (no error)"=w189) -> ("error out"=w188:errorcluster)  [unwired: 5 in, 1 out]
  n356 = invoke class="VI" method="FP.Close"(reference=w41, error in=w188) -> (error out=→"error out":errorcluster)  [unwired: 1 in, 2 out]
